vi "rpc_tsmaster_cmd_write_system_var.vi"(6 "AValue":string, 8 "error in (no error)":errorcluster caption="Incorrect input (no errors)", 9 "AHandle":i32, 10 "ACompleteName":string, 11 "Path input":path) -> (0 "error output":errorcluster, 1 "AHandle out":i32, 2 "return":i32, 3 "Path output":path)   [LabVIEW 2014]
doc: "Function introduction: Write system variables by name from remote TSMaster\nAfter calling the location to create TSMaster Rpc client\nInput parameter AHHandle: TSMaster Rpc client handle\nACompleteName: System variable name\nAValue: Data Value\nReturn value==0: Function execution successful"
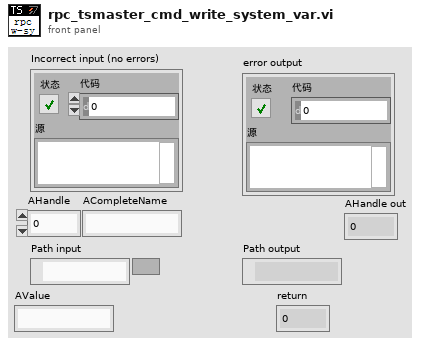
[diagram p1: front panel]
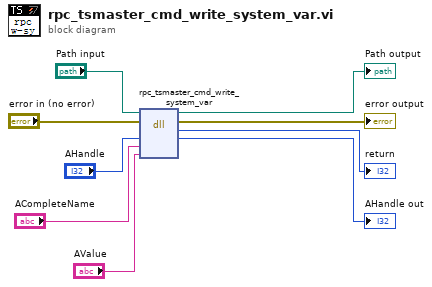
[diagram p0: block diagram]
diagram:
  n1 = dll-call lib="C:/Program Files (x86)/TOSUN/TSMaster12/TSMaster/bin/TSMaster.dll" fn="rpc_tsmaster_cmd_write_system_var"(path in="Path input", error in="error in (no error)", "AHandle"="AHandle", "ACompleteName"="ACompleteName", "AValue"="AValue") -> (path out=→"Path output":path, error out=→"error output":errorcluster, "返回类型"=→"return":i32, "AHandle"=→"AHandle out":i32)  [unwired: 3 in]
